vi "Draw Workspace.vi"(7 "name":string, 8 "error in (no error)":errorcluster, 9 "workspace in":dbl[][](array[numeric]), 10 "parent sence":refnum<vi>, 11 "Delta Analyzor in":refnum<class "Delta Analyzor.lvclass">) -> (0 "error out":errorcluster, 1 "Wrkspc Obj":refnum<vi>, 2 "parent sence out":refnum<vi>, 3 "Delta Analyzor out":refnum<class "Delta Analyzor.lvclass">)   [LabVIEW 2013, in "Delta Analyzor.lvclass"]
uses:
  Delta Analyzor.lvclass
  <vilib>/Utility/miscctls.llb/LV3DPointTypeDef.ctl
  <vilib>/Utility/miscctls.llb/LVRGBAColorTypeDef.ctl
  <vilib>/picture/3D Picture Control/Object/Create Object (name).vi
  <vilib>/picture/3D Picture Control/NI_3D Picture Control.lvlib
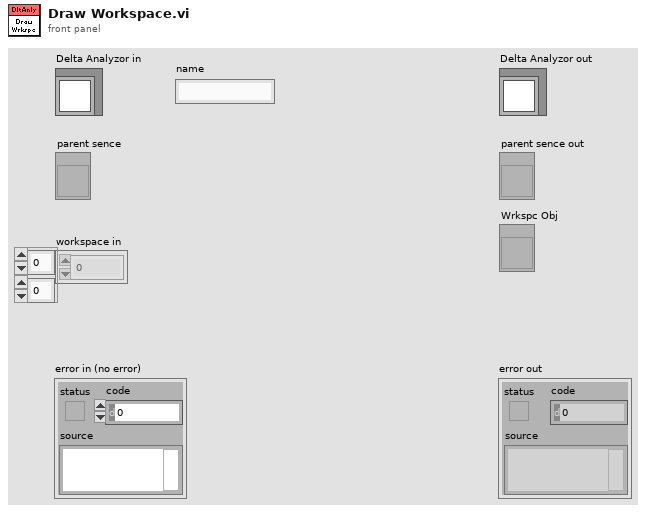
[diagram p1: front panel]
types:
  T1 = typedef "LV3DPointTypeDef.ctl" = cluster{"X":sgl, "Y":sgl, "Z":sgl}
  T2 = enum16{"Overall", "Per Primitive", "Per Vertex", "Binding Off"}
  T3 = enum16{"Points", "Lines", "Line Strip", "Line Loop", "Triangles", "Triangle Strip", "Triangle Fan", "Quads", "Quad Strip", "Polygon"}
  T4 = typedef "LVRGBAColorTypeDef.ctl" = cluster{"Red":sgl, "Green":sgl, "Blue":sgl, "Alpha":sgl}
  T5 = cluster{"workspace in[0]":dbl, "workspace in[1]":dbl, "workspace in[2]":dbl}
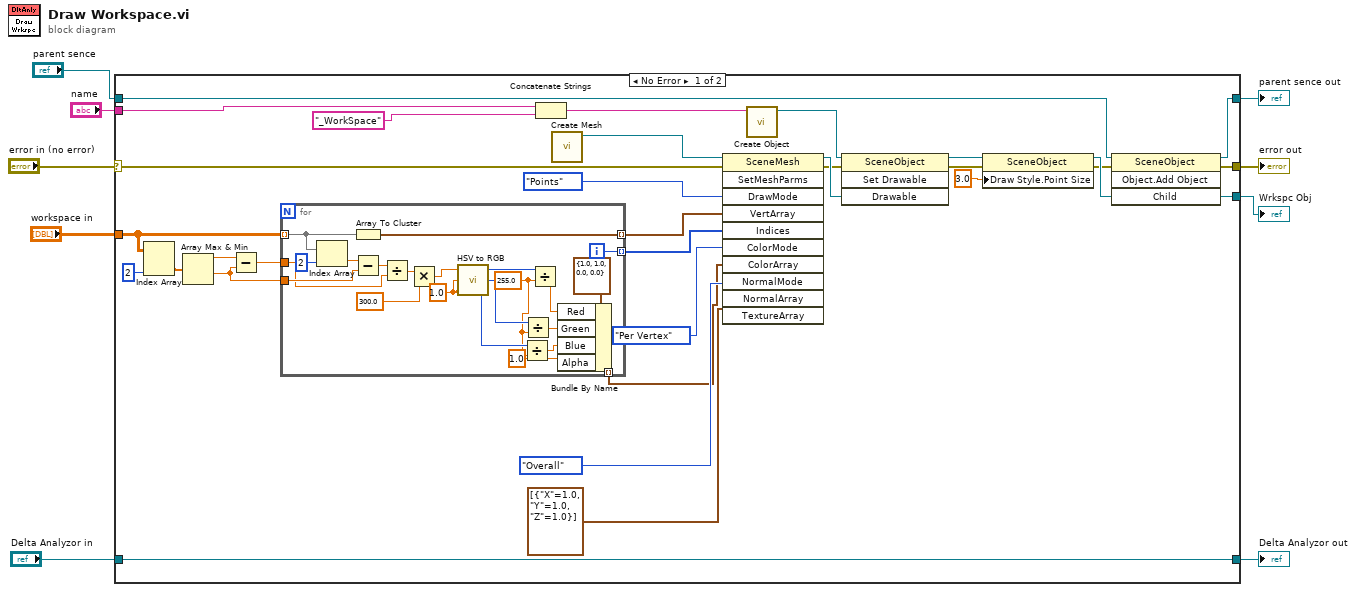
[diagram p0: block diagram]
diagram:
  n1 = case shown="No Error" "error in (no error)" {
    selector: "error in (no error)" -> [w18 w65]
    tunnel: [w17 w65] -> w8
    tunnel: [w40 w64] -> w6
    tunnel: "Delta Analyzor in" -> [w40 w64]
    tunnel: "parent sence" -> [w30 w63]
    tunnel: "name" -> [w39 _]
    tunnel: "workspace in" -> [w16 _]
    tunnel: [w29 _] -> w2
    tunnel: [w28 w63] -> w1
    frame No Error {
      n2 = Index Array(array=w16, index (col)=2 ("disabled index (col)")) -> (element=w14:dbl[])  [unwired: 1 in]
      n3 = Array Max & Min(array=w14) -> (max value=w13:dbl, min value=w11:dbl)  [unwired: 2 out]
      n4 = Subtract(x=w13, y=w11) -> (x-y=w12:dbl)
      n5 = for {
        tunnel: w16 -> [w60] mode=indexing
        tunnel: [w62] -> w34 mode=indexing
        tunnel: [w61] -> w25 mode=indexing
        tunnel: w12 -> [w55]
        tunnel: w11 -> [w57]
        tunnel: [w41] -> w10 mode=indexing
        i -> [w61]
        w44 = 255.0
        w54 = 1.0 ("S")
        n6 = Index Array(array=w60, index=2) -> (element=w58:dbl)
        n7 = Array To Cluster(array=w60) -> (cluster=w62:T5)
        n8 = Subtract(x=w58, y=w57) -> (x-y=w56:dbl)
        n9 = Divide(x=w56, y=w55) -> (x/y=w53:dbl)
        n10 = Multiply(x=w53, y=300.0) -> (x*y=w51:dbl)
        n11 = call "HSV to RGB.vi"("V"=w54, "S"=w54, "H"=w51) -> ("B"=w45:u8, "G"=w47:u8, "R"=w49:u8)
        n12 = Divide(x=w45, y=w44) -> (x/y=w43:dbl)
        n13 = Divide(x=w47, y=w44) -> (x/y=w46:dbl)
        n14 = Divide(x=w49, y=w44) -> (x/y=w48:dbl)
        n15 = Bundle By Name(cluster=T4 {"Red"=1.0, "Green"=1.0, "Blue"=0.0, "Alpha"=0.0} ("Color"), "Red"=w48, "Green"=w46, "Blue"=w43, "Alpha"=sgl 1.0) -> (w41:T4)
      }
      n16 = Concatenate Strings(w39, "_WorkSpace" ("string")) -> (w37:string)
      n17 = call <vilib>:"Create Mesh.vi"() -> ("New Mesh Refnum"=w36:refnum<vi>)  [unwired: 10 in, 1 out]
      n18 = invoke class="SceneMesh" method="SetMeshParms"(reference=w36, error in=w18, "DrawMode"=T3."Points" ("Draw Mode"), "VertArray"=w34, "Indices"=w25, "ColorMode"=T2."Per Vertex" ("Color Binding Mode"), "ColorArray"=w10, "NormalMode"=T2."Overall" ("Normal Binding Mode"), "NormalArray"=T1[] [{"X"=1.0, "Y"=1.0, "Z"=1.0}] ("Normal Array")) -> (reference out=w31:refnum<vi>, error out=w21:errorcluster)  [unwired: 2 in, 9 out]
      n19 = call-poly <vilib>:"Create Object.vi"("Name"=w37) -> ("Scene:New Object"=w32:refnum<vi>)  [unwired: 9 in, 1 out]
      n20 = invoke class="SceneObject" method="Set Drawable"(reference=w32, error in=w21, "Drawable"=w31) -> (reference out=w24:refnum<vi>, error out=w20:errorcluster)  [unwired: 1 in, 2 out]
      n21 = property class="SceneObject"(reference=w24, error in=w20, "Draw Style.Point Size"=sgl 3.0 ("Draw Style:Point Size")) -> (reference out=w22:refnum<vi>, error out=w19:errorcluster)
      n22 = invoke class="SceneObject" method="Object.Add Object"(reference=w30, error in=w19, "Child"=w22) -> (reference out=w28:refnum<vi>, error out=w17:errorcluster, "Child"=w29:refnum<vi>)  [unwired: 1 in, 1 out]
    }
    frame Error {
    }
  }
  "error out" <- w8
  "Delta Analyzor out" <- w6
  "Wrkspc Obj" <- w2
  "parent sence out" <- w1
